vi "API - Continuous Capture - Capture Single Buffer.vi"(8 "error in":errorcluster, 9 "Data Size":T1, 10 "Buffer Block Size (Samples/Channel)":i32=256, 11 "configuration file path":path) -> (0 "error out":errorcluster)   [LabVIEW 2017, in "DTACQ - Network Enabled Device Driver.lvlib"]
doc: "Captures a single buffer length of waveform data, using the continuous capture mode"
uses:
  DTACQ - Network Enabled Device Driver.lvlib
  Communications/Typedefs/Data Size--Enum.ctl
  Close Continuous Mode.vi
  Read Continuous Data and Write to Shared Variable.vi
  Initialise Continuous Capture Mode.vi
  Communications/Communications Library.lvlib
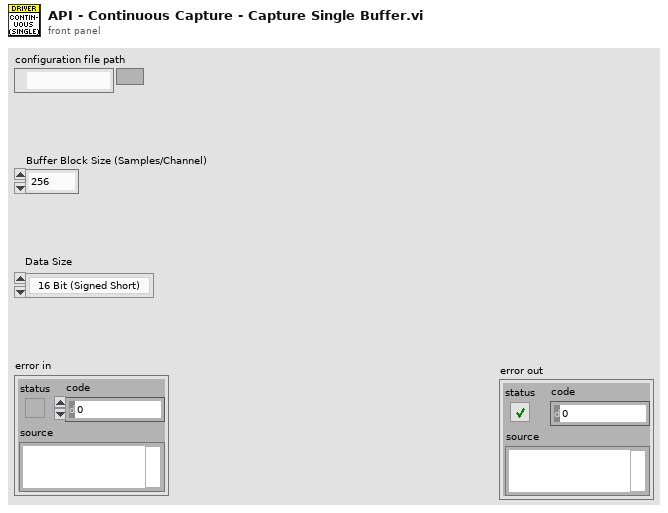
[diagram p1: front panel]
types:
  T1 = typedef "Communications Library.lvlib/Data Size--Enum.ctl" = enum16{"16 Bit (Signed Short)", "32 Bit (Signed Long)"}
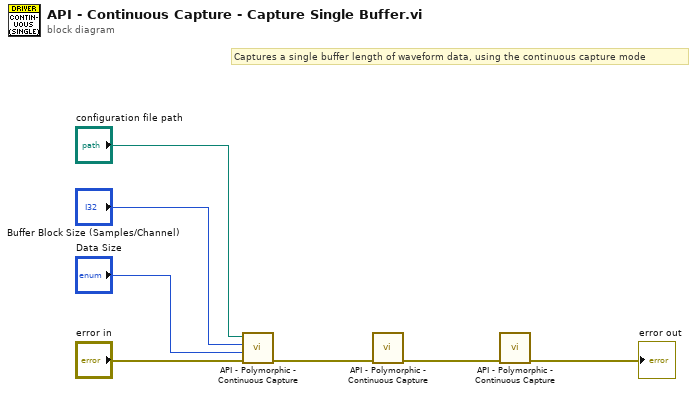
[diagram p0: block diagram]
diagram:
  # "Captures a single buffer length of waveform data, using the continuous capture mode"
  n1 = call-poly "API - Polymorphic - Continuous Capture.vi"("error in"="error in", "Data Size"="Data Size", "Buffer Block Size (Samples/Channel)"="Buffer Block Size (Samples/Channel)", "configuration file path"="configuration file path") -> ("error out"=w3:errorcluster)  [unwired: 7 in]
  n2 = call-poly "API - Polymorphic - Continuous Capture.vi"("error in"=w3) -> ("error out"=w2:errorcluster)  [unwired: 10 in]
  n3 = call-poly "API - Polymorphic - Continuous Capture.vi"("error in"=w2) -> ("error out"=→"error out":errorcluster)  [unwired: 10 in]
